vi "Calculate DNL.vi"(0 "Deviated Values":dbl[](array[numeric]), 11 "Error in":errorcluster) -> (4 "Codes":dbl[](array[numeric]), 6 "DNL Values":dbl[](array[numeric]), 15 "Error out":errorcluster)   [LabVIEW 2020, in "INL DNL Test.lvclass"]
doc: "Calculate DNL for the deviated values"
uses:
  INL DNL Test.lvclass
  INL DNL Test.lvclass/INL DNL Test.ctl
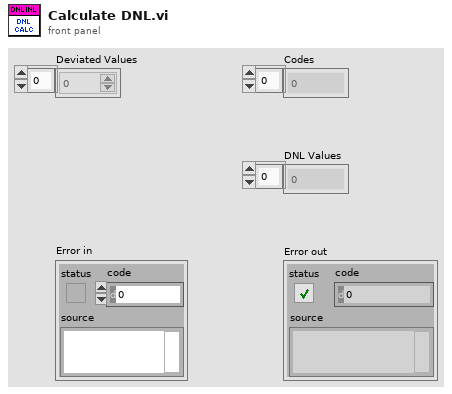
[diagram p1: front panel]
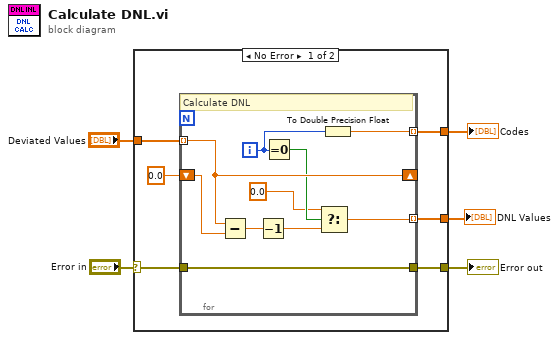
[diagram p0: block diagram]
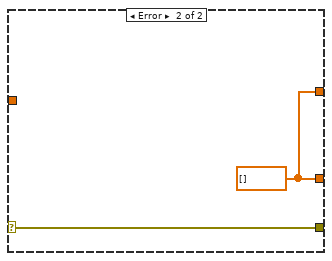
[diagram p2: hidden frame]
diagram:
  n1 = case shown="No Error" "Error in" {
    selector: "Error in" -> [w8 w23]
    tunnel: "Deviated Values" -> [w10 _]
    tunnel: [w9 w22] -> w4
    tunnel: [w7 w23] -> w2
    tunnel: [w6 w22] -> w1
    frame No Error {
      n2 = for {
        tunnel: w10 -> [w21] mode=indexing
        shift-right: [w21] -> _
        shift-left: 0.0 ("Error rate 2") -> [w20]
        tunnel: [w16] -> w9 mode=indexing
        tunnel: [w14] -> w7
        tunnel: w8 -> [w14]
        tunnel: [w12] -> w6 mode=indexing
        i -> [w13]
        # "Calculate DNL"
        n3 = Subtract(x=w21, y=w20) -> (x-y=w17:dbl)
        n4 = Decrement(x=w17) -> (x-1=w15:dbl)
        n5 = Equal To 0?(x=w13) -> (x = 0?=w19:bool)
        n6 = Select(t=0.0, s=w19, f=w15) -> (s? t:f=w16:dbl)
        n7 = To Double Precision Float(number=w13) -> (double precision float=w12:dbl)
      }
    }
    frame Error {
      w22 = dbl[] []
    }
  }
  "DNL Values" <- w4
  "Error out" <- w2
  "Codes" <- w1
